vi "test_9215_9264.vi"() -> ()   [LabVIEW 2014]
uses:
  <vilib>/rvi/Emulation/niFpgaGetClockAttributes.vi
  <vilib>/rvi/Emulation/niFpgaSctlEmulationGetInTimedLoop.vi
  <vilib>/rvi/Emulation/niFpgaEmulationReportErrorSimple.vi
  <vilib>/rvi/Emulation/niFpgaProcessEmulError.vi
  <vilib>/rvi/eio/common/nirviEmuTemplateMethod_errors.vi
  <vilib>/rvi/Emulation/niFpgaCriticalErrorInLSC.vi
  <vilib>/rvi/interface/RandomDataEmulation/nirviRandomDataMultiElementFPGAFIFO.vi
  <instcachedir>/0/nirviRandomDataMultiElementFPGAFIFO_AD0CFC12EF974623A9C2E4184BC062B2.lvgen/nirviRandomDataMultiElementFPGAFIFO_AD0CFC12EF974623A9C2E4184BC062B2_023.vi
  <vilib>/rvi/interface/RandomDataEmulation/niFpgaRandomDataHandleErrors.vi
  <vilib>/eio/EIONode/EIONode.xnode
  <vilib>/rvi/DataTransferAndStorage/Container/XNode/niFpgaContainer.xnode
  <vilib>/rvi/interface/RandomDataEmulation/nirviRandomDataFpgaMultiElementTemplate.vi
panel:
  in  "OP_y":fxp<+/-,32,8>
  in  "OP_p":fxp<+/-,32,8>
  out "Strain_dc_p":fxp<+/-,20,5>
  out "Strain_dc_y":fxp<+/-,20,5>
  out "Strain_y_Avg2":fxp<+/-,30,3>
  out "Strain_y_Avg4":fxp<+/-,31,3>
  out "Strain_y_Avg8":fxp<+/-,32,4>
  out "Strain_p_Avg2":fxp<+/-,30,3>
  out "Strain_p_Avg4":fxp<+/-,31,3>
  out "Strain_p_Avg8":fxp<+/-,32,4>
  out "Mod3/AI2":fxp<+/-,32,6>
  out "Mod3/AI1":fxp<+/-,32,6>
  in  "Strain zero_y":bool
  in  "Strain zero_p":bool
  in  "Sampling Rate (uSec)":u32 caption="Sampling Rate (mSec)"
  out "Raw_y":fxp<+/-,32,6>
  out "Raw_p":fxp<+/-,32,6>
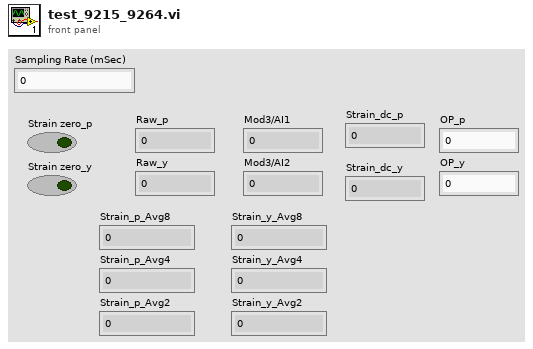
[diagram p1: front panel]
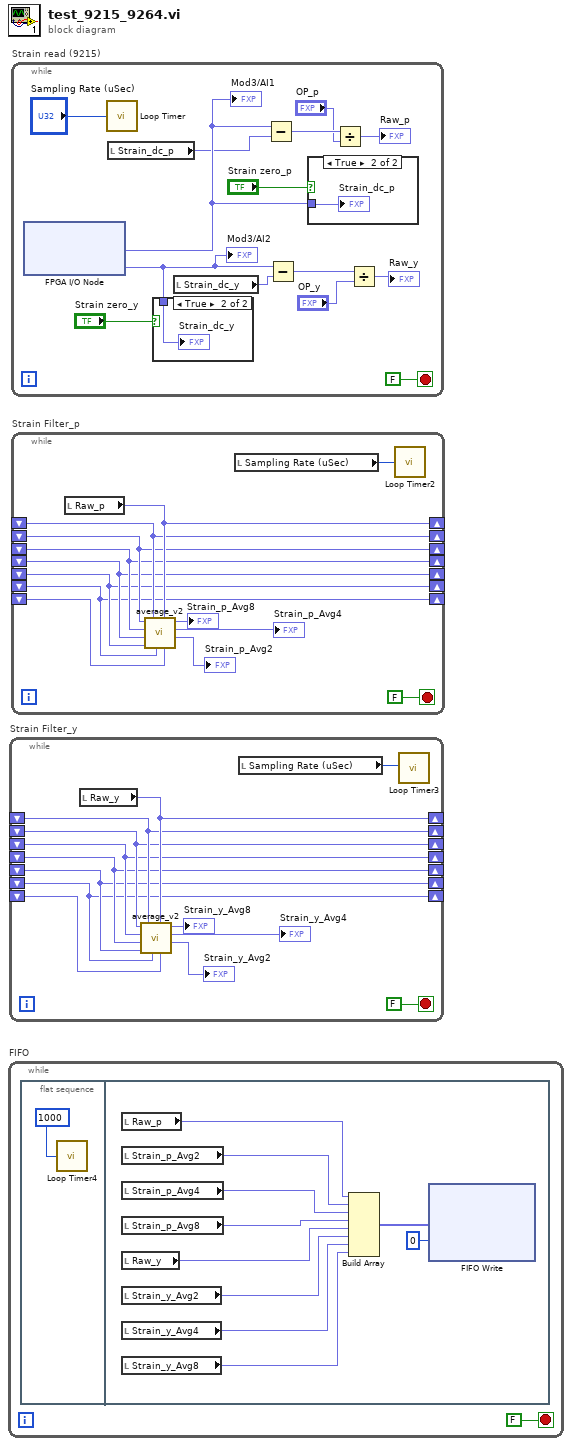
[diagram p0: block diagram]
diagram:
  n1 = while "FIFO" {
    stop <- FALSE stop-if-true
    n2 = flat-sequence {
      frame #0 {
        n3 = call "Loop Timer4"("Count(uSec)"=u32 1000 ("Count(mSec)")) -> ()  [unwired: 1 out]
      }
      frame #1 {
        n4 = local read "Raw_p"() -> (w10:fxp<+/-,32,6>)
        n5 = local read "Strain_p_Avg2"() -> (w9:fxp<+/-,30,3>)
        n6 = local read "Strain_p_Avg4"() -> (w8:fxp<+/-,31,3>)
        n7 = local read "Strain_p_Avg8"() -> (w7:fxp<+/-,32,4>)
        n8 = local read "Raw_y"() -> (w6:fxp<+/-,32,6>)
        n9 = local read "Strain_y_Avg2"() -> (w5:fxp<+/-,30,3>)
        n10 = local read "Strain_y_Avg4"() -> (w4:fxp<+/-,31,3>)
        n11 = local read "Strain_y_Avg8"() -> (w3:fxp<+/-,32,4>)
        n12 = Build Array(w10, w9, w8, w7, w6, w5, w4, w3) -> (w11:fxp<+/-,34,6>[])
        n13 = xnode ("FIFO Write")("Element"=w11, "Timeout"=0) -> ()  [unwired: 1 in, 2 out]
      }
    }
  }
  n14 = while "Strain Filter_y" {
    shift-right: [w24] -> _
    shift-left: _ -> [w23]
    shift-right: [w23] -> _
    shift-left: _ -> [w22]
    shift-right: [w22] -> _
    shift-left: _ -> [w21]
    shift-right: [w21] -> _
    shift-left: _ -> [w20]
    shift-right: [w20] -> _
    shift-left: _ -> [w19]
    shift-right: [w19] -> _
    shift-left: _ -> [w18]
    shift-right: [w18] -> _
    shift-left: _ -> [w17]
    stop <- FALSE stop-if-true
    n15 = local read "Raw_y"() -> (w24:fxp<+/-,32,6>)
    n16 = call "average_v2.vi"("Numeric 8"=w17, "Numeric"=w24, "Numeric 7"=w18, "Numeric 2"=w23, "Numeric 6"=w19, "Numeric 5"=w20, "Numeric 4"=w21, "Numeric 3"=w22) -> ("Mean (2pt)"=→"Strain_y_Avg2":fxp<+/-,30,3>, "Mean (4pt)"=→"Strain_y_Avg4":fxp<+/-,31,3>, "Mean (8pt)"=→"Strain_y_Avg8":fxp<+/-,32,4>)  [unwired: 1 in]
    n17 = local read "Sampling Rate (uSec)"() -> (w25:u32)
    n18 = call "Loop Timer3"("Count(uSec)"=w25) -> ()  [unwired: 1 out]
  }
  n19 = while "Strain read (9215)" {
    stop <- FALSE stop-if-true
    n20 = xnode "FPGA I/O Node"() -> ("Mod3/AI1"=w34:fxp<+/-,20,5>, "Mod3/AI2"=w37:fxp<+/-,20,5>)  [unwired: 2 in, 2 out]
    "Mod3/AI1" <- w34
    "Mod3/AI2" <- w37
    n21 = call "Loop Timer"("Count(uSec)"="Sampling Rate (uSec)") -> ()  [unwired: 1 out]
    n22 = local read "Strain_dc_p"() -> (w33:fxp<+/-,20,5>)
    n23 = case shown="True" "Strain zero_y" {
      tunnel: w37 -> [_ w41]
      frame False {
      }
      frame True {
        "Strain_dc_y" <- w41
      }
    }
    n24 = local read "Strain_dc_y"() -> (w36:fxp<+/-,20,5>)
    n25 = Subtract(x=w34, y=w33) -> (x-y=w30:fxp<+/-,32,6>)
    n26 = Subtract(x=w37, y=w36) -> (x-y=w27:fxp<+/-,32,6>)
    n27 = case shown="True" "Strain zero_p" {
      tunnel: w34 -> [_ w40]
      frame False {
      }
      frame True {
        "Strain_dc_p" <- w40
      }
    }
    n28 = Divide(x=w30, y="OP_p") -> (x/y=→"Raw_p":fxp<+/-,64,31>)
    n29 = Divide(x=w27, y="OP_y") -> (x/y=→"Raw_y":fxp<+/-,64,31>)
  }
  n30 = while "Strain Filter_p" {
    shift-right: [w52] -> _
    shift-left: _ -> [w51]
    shift-right: [w51] -> _
    shift-left: _ -> [w50]
    shift-right: [w50] -> _
    shift-left: _ -> [w49]
    shift-right: [w53] -> _
    shift-left: _ -> [w52]
    shift-right: [w49] -> _
    shift-left: _ -> [w48]
    shift-right: [w48] -> _
    shift-left: _ -> [w47]
    shift-right: [w47] -> _
    shift-left: _ -> [w46]
    stop <- FALSE stop-if-true
    n31 = local read "Raw_p"() -> (w53:fxp<+/-,32,6>)
    n32 = call "average_v2.vi"("Numeric 8"=w46, "Numeric"=w53, "Numeric 7"=w47, "Numeric 2"=w52, "Numeric 6"=w48, "Numeric 5"=w49, "Numeric 4"=w50, "Numeric 3"=w51) -> ("Mean (2pt)"=→"Strain_p_Avg2":fxp<+/-,30,3>, "Mean (4pt)"=→"Strain_p_Avg4":fxp<+/-,31,3>, "Mean (8pt)"=→"Strain_p_Avg8":fxp<+/-,32,4>)  [unwired: 1 in]
    n33 = local read "Sampling Rate (uSec)"() -> (w54:u32)
    n34 = call "Loop Timer2"("Count(uSec)"=w54) -> ()  [unwired: 1 out]
  }
